vi "ReadListFGV.vi"(7 "Set":bool, 8 "SendData":string, 9 "Data":string, 10 "アドレス":string, 11 "Read Data":T2(array[cluster])) -> (2 "空?":bool, 3 "Read List Out":T2(array[cluster]), 4 "Read Log":T1(array[cluster]))   [LabVIEW 2021]
doc: "受信したデータと、送り元のアドレス、直前に送信したデータのクラスターのリストを保持します。\nこのリストに登録したデータは処理されて必要な情報を利用します。"
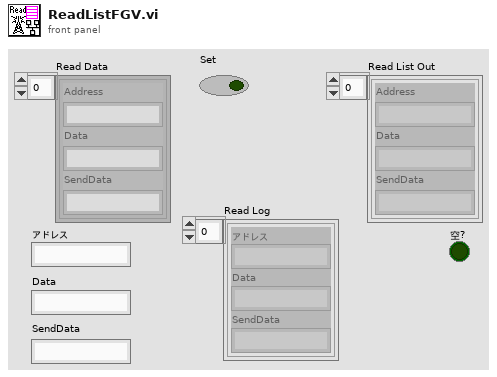
[diagram p1: front panel]
types:
  T1 = cluster{"アドレス":string, "Data":string, "SendData":string}[]
  T2 = cluster{"Address":string, "Data":string, "SendData":string}[]
  T3 = cluster{"アドレス":string, "Data":string, "SendData":string}
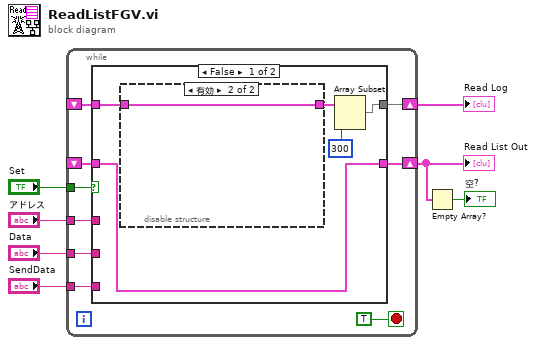
[diagram p0: block diagram]
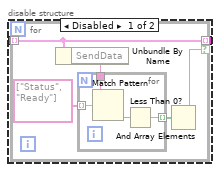
[diagram p2: hidden frame]
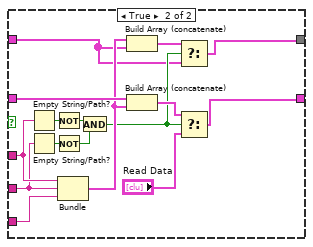
[diagram p3: hidden frame]
diagram:
  n1 = while {
    tunnel: "アドレス" -> [w14]
    tunnel: "Data" -> [w13]
    shift-right: [w16] -> w6
    shift-left: _ -> [w15]
    tunnel: "Set" -> [w11]
    tunnel: "SendData" -> [w10]
    shift-right: [w8] -> w1
    shift-left: _ -> [w9]
    stop <- TRUE stop-if-true
    n2 = case shown="False" w11 {
      tunnel: [w21 w47] -> w16
      tunnel: w15 -> [w21 w49]
      tunnel: w14 -> [_ w45]
      tunnel: w13 -> [_ w42]
      tunnel: w10 -> [_ w39]
      tunnel: w9 -> [w18 w34]
      tunnel: [w19 w35] -> w8
      frame False {
        n3 = disable-structure shown="有効" {
          disable-tunnel: w18 -> [w23 w33]
          disable-tunnel: [w22 w33] -> w17
          frame Disabled {
            n4 = for {
              tunnel: w23 -> [w28] mode=indexing
              tunnel: [w28] -> w22 mode=indexing if=w24
              n5 = Unbundle By Name(w28) -> ("SendData"=w27:string)
              n6 = for {
                tunnel: w27 -> [w32]
                tunnel: string[] ["Status", "Ready"] ("正規表現") -> [w31] mode=indexing
                tunnel: [w29] -> w25 mode=indexing
                n7 = Match Pattern(string=w32, regular expression=w31) -> (offset past match=w30:i32)  [unwired: 1 in, 3 out]
                n8 = Less Than 0?(x=w30) -> (x < 0?=w29:bool)
              }
              n9 = And Array Elements(Boolean array=w25) -> (logical AND=w24:bool)
            }
          }
          frame Enabled {
          }
        }
        n10 = Array Subset(array=w17, length=300 ("長さ")) -> (w19:T1)  [unwired: 1 in]
      }
      frame True {
        n11 = Empty String/Path?(string/path=w45) -> (empty?=w44:bool)
        n12 = Empty String/Path?(string/path=w42) -> (empty?=w41:bool)
        n13 = Not(x=w44) -> (.not. x?=w43:bool)
        n14 = Not(x=w41) -> (.not. x?=w40:bool)
        n15 = Bundle("アドレス"=w45, "Data"=w42, "SendData"=w39) -> (w38:T3)  [unwired: 1 in]
        n16 = And(x=w43, y=w40) -> (x .and. y?=w37:bool)
        n17 = Build Array (concatenate)(w38, w34) -> (w36:T1)
        n18 = Build Array (concatenate)(w49, w38) -> (w48:T1)
        n19 = Select(t=w36, s=w37, f=w34) -> (s? t:f=w35:T1)
        n20 = Select(t=w48, s=w37, f="Read Data") -> (s? t:f=w47:T2)
      }
    }
  }
  "Read List Out" <- w6
  "Read Log" <- w1
  n21 = Empty Array?(array=w6) -> (empty?=→"空?":bool)
